vi "Limit entered trial length.vi"(8 "error in (no error)":errorcluster) -> (0 "error out":errorcluster)   [LabVIEW 2017]
uses:
  ROI Entry screen/Globals/gl_ROI Entry UI globals.vi
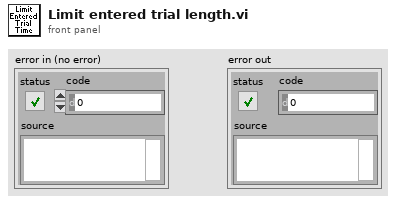
[diagram p1: front panel]
types:
  T1 = typedef "ROI ID Enum.ctl" = enum16{"Point", "MiniScan", "Comp. MiniScan", "Rectangle", "Comp. volume", "Arb. plane point"}
  T2 = typedef "ROI entry screen ctrl refs cluster.ctl" = cluster{"Done button":refnum<vi>, "Imaging button":refnum<vi>, "Acquisition button":refnum<vi>, "POI dwell time (us)":refnum<vi>, "Scan dwell time per pixel (us)":refnum<vi>, "# of planes":refnum<vi>, "Zoom Ctrl":refnum<vi>, "Equal size":refnum<vi>, "Channel":refnum<vi>, "Image Display":refnum<vi>, "Z-Plane Selector":refnum<vi>, "Number of lines left":refnum<vi>, "Z-stack folder path":refnum<vi>, "POI Density":refnum<vi>, "Arb Plane Entry":refnum<vi>, "Whole plane":refnum<vi>, "Clear Last":refnum<vi>, "Clear All":refnum<vi>, "Trial Length (sec)":refnum<vi>, "Palette Type":refnum<vi>, "Intensity slider":refnum<vi>, "# POI":refnum<vi>, "Max Z Proj":refnum<vi>, "Zplane ind":refnum<vi>, "Wavelength (nm)":refnum<vi>, "Number of Trials":refnum<vi>, "Funct stim.trig.enable":refnum<vi>, "Funct stim.trig.delay (s)":refnum<vi>, "Line Mode":refnum<vi>, "Step size (µm)":refnum<vi>, "ROI move mode":refnum<vi>, "Cool-down time (s)":refnum<vi>, "Enable cool-down time":refnum<vi>, "Motor Z ind. (um)":refnum<vi>, "AOL Z ind. (um)":refnum<vi>, "Load Reference Image":refnum<vi>}
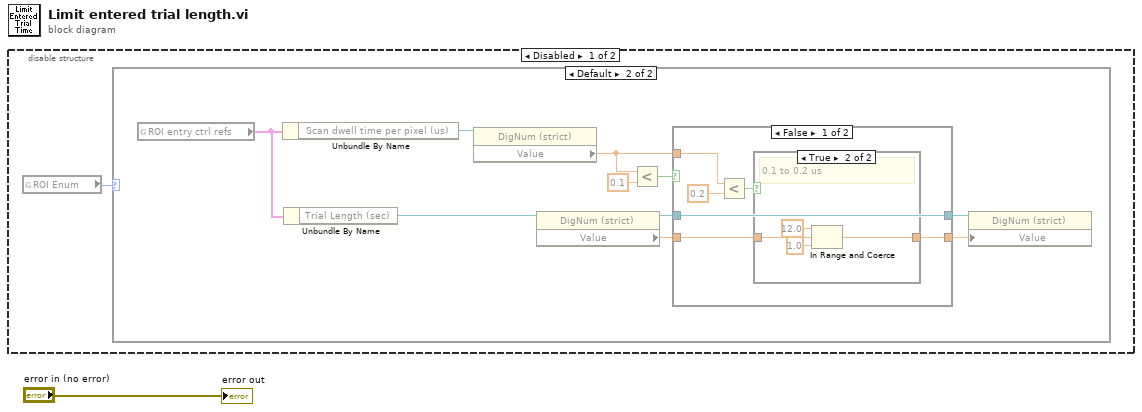
[diagram p0: block diagram]
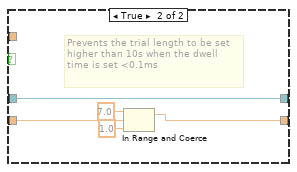
[diagram p4: hidden frame]
diagram:
  n1 = disable-structure shown="Disabled" {
    frame Disabled {
      n2 = global read "gl_ROI Entry UI globals.vi" "ROI Enum"() -> (w2:T1)
      n3 = case shown="Default" w2 {
        frame "Point" {
        }
        frame Default {
          n4 = global read "gl_ROI Entry UI globals.vi" "ROI entry ctrl refs"() -> (w4:T2)
          n5 = Unbundle By Name(w4) -> ("Scan dwell time per pixel (us)"=w5:refnum<vi>)
          n6 = Unbundle By Name(w4) -> ("Trial Length (sec)"=w10:refnum<vi>)
          n7 = property class="DigNum (strict)"(reference=w5) -> ("Value"=w3:dbl)  [unwired: 1 in, 2 out]
          n8 = property class="DigNum (strict)"(reference=w10) -> (reference out=w11:refnum<vi>, "Value"=w12:dbl)  [unwired: 1 in, 1 out]
          n9 = Less?(x=w3, y=0.1) -> (x < y?=w7:bool)
          n10 = case shown="False" w7 {
            tunnel: w11 -> [w18 w25]
            tunnel: [w18 w25] -> w8
            tunnel: [w17 w26] -> w9
            tunnel: w12 -> [w16 w24]
            tunnel: w3 -> [w14 _]
            frame False {
              n11 = Less?(x=w14, y=0.2) -> (x < y?=w13:bool)
              n12 = case shown="True" w13 {
                tunnel: [w19 w21] -> w17
                tunnel: w16 -> [w19 w20]
                frame False {
                  # "Limited by the\ncontrol numerical\nentry itself, to the \nuser-configurable limit\nin the global."
                  # ">0.2us"
                }
                frame True {
                  # "0.1 to 0.2 us"
                  n13 = In Range and Coerce(upper limit=12.0, x=w20, lower limit=1.0) -> (coerced(x)=w21:dbl)  [unwired: 1 out]
                }
              }
            }
            frame True {
              # "Prevents the trial length to be set higher than 10s when the dwell time is set <0.1ms"
              n14 = In Range and Coerce(upper limit=7.0, x=w24, lower limit=1.0) -> (coerced(x)=w26:dbl)  [unwired: 1 out]
            }
          }
          n15 = property class="DigNum (strict)"(reference=w8, "Value"=w9) -> ()  [unwired: 1 in, 2 out]
        }
      }
    }
    frame Enabled {
    }
  }
  "error out" <- "error in (no error)"
